vi "Get RDMA Error Info.vi"(11 "error":T1=enum."Too Many Transfers") -> (2 "description":string, 3 "code":i32)   [LabVIEW 2020, in "RDMA.lvlib" / "RDMA Transceiver.lvclass"]
uses:
  RDMA Transceiver.lvclass
  Errors.ctl
  Base Error Code.vi
  RDMA Transceiver.lvclass/RDMA Transceiver.ctl
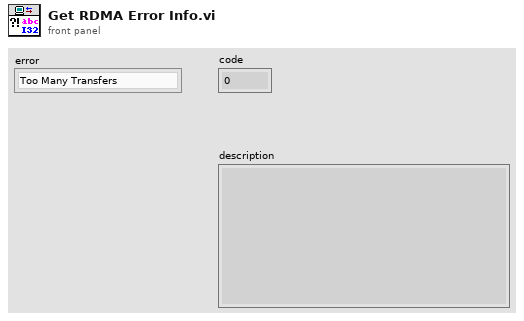
[diagram p1: front panel]
types:
  T1 = typedef "RDMA.lvlib/RDMA Transceiver.lvclass/Errors.ctl" = enum16{"Invalid RDMA Configuration", "Too Many Transfers", "Size Mismatch", "Unknown Setting"}
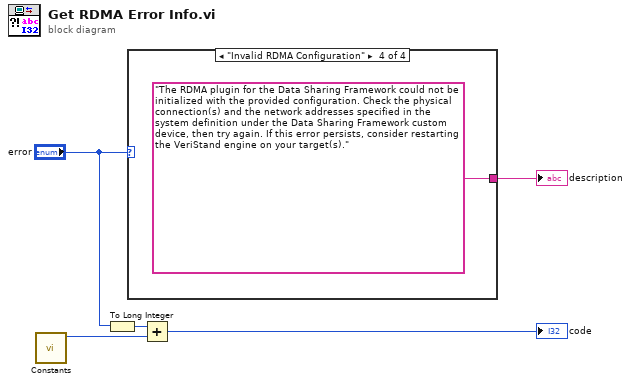
[diagram p0: block diagram]
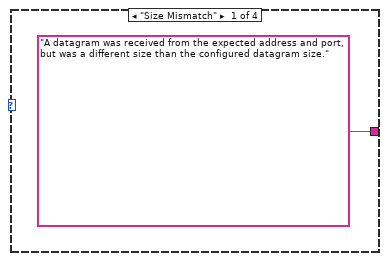
[diagram p2: hidden frame]
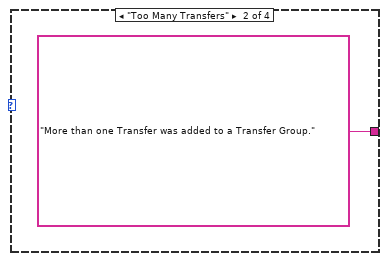
[diagram p3: hidden frame]
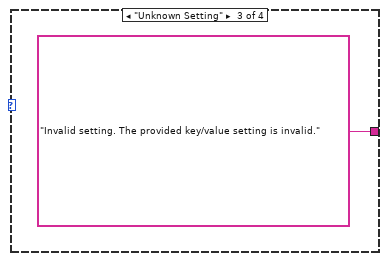
[diagram p4: hidden frame]
diagram:
  n1 = call-poly "Constants.vi"() -> ("base error code"=w5:i32)  [unwired: 11 in]
  n2 = To Long Integer(number="error") -> (32bit integer=w4:i32)
  n3 = case shown="\"Invalid RDMA Configuration\"" "error" {
    tunnel: ["A datagram was received from the expected address and port, but was a different size than the configured datagram size." "More than one Transfer was added to a Transfer Group." "Invalid setting. The provided key/value setting is invalid." "The RDMA plugin for the Data Sharing Framework could not be initialized with the provided configuration. Check the physical connection(s) and the network addresses specified in the system definition under the Data Sharing Framework custom device, then try again. If this error persists, consider restarting the VeriStand engine on your target(s)."] -> w1
    frame "Size Mismatch" {
    }
    frame "Too Many Transfers" {
    }
    frame "Unknown Setting" {
    }
    frame "Invalid RDMA Configuration" {
    }
  }
  "description" <- w1
  n4 = Add(x=w4, y=w5) -> (x+y=→"code":i32)
